vi "ex3.vi"() -> ()   [LabVIEW 2019]
panel:
  in  "stop":bool
  out "Array":bool[](array[boolean])
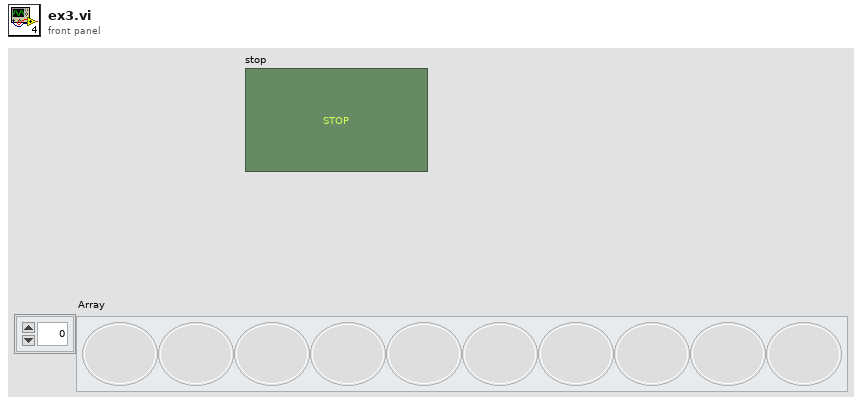
[diagram p1: front panel]
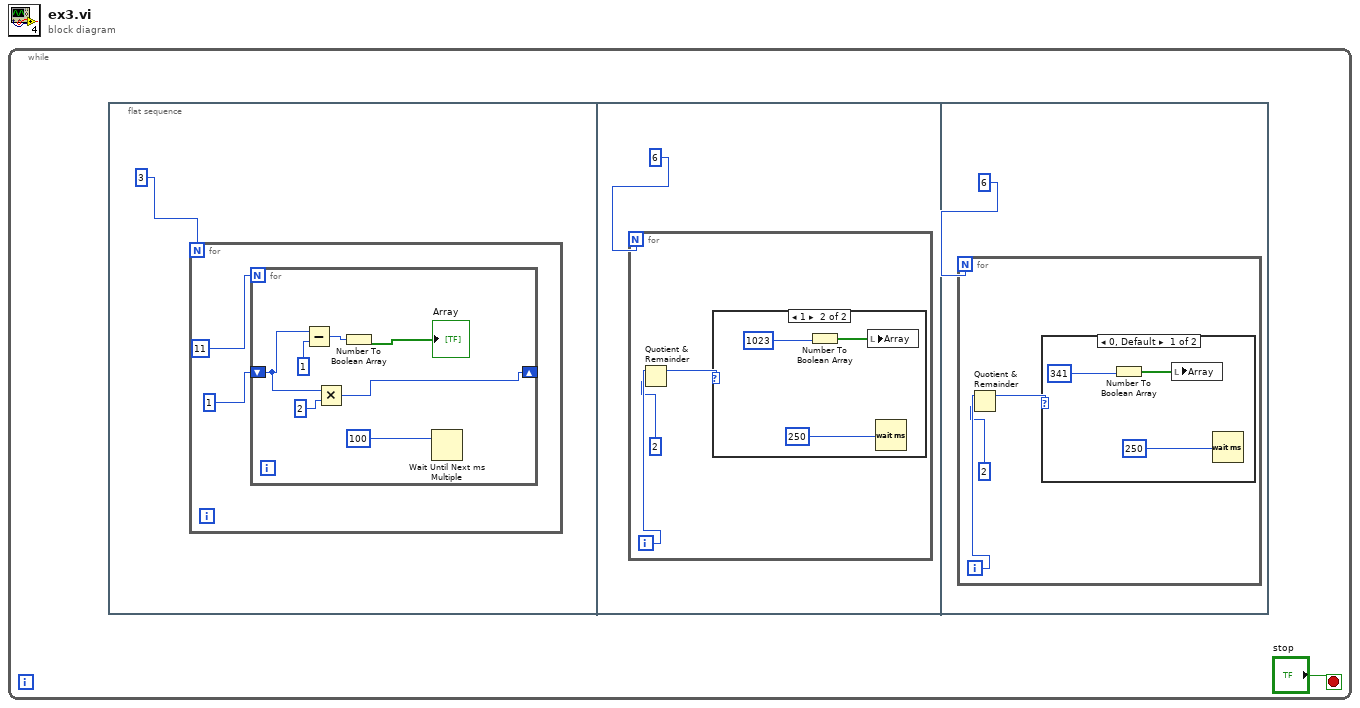
[diagram p0: block diagram]
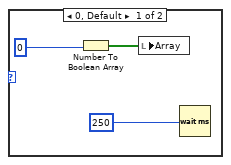
[diagram p2: hidden frame]
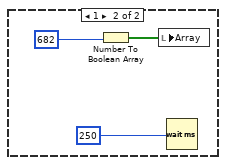
[diagram p3: hidden frame]
diagram:
  n1 = while {
    stop <- "stop" stop-if-true
    n2 = flat-sequence {
      frame #0 {
        n3 = for {
          N: 3 -> [_]
          n4 = for {
            N: 11 -> [_]
            shift-right: [w8] -> _
            shift-left: 1 -> [w5]
            n5 = Subtract(x=w5, y=1) -> (x-y=w7:i32)
            n6 = Multiply(x=w5, y=2) -> (x*y=w8:i32)
            n7 = Number To Boolean Array(number=w7) -> (Boolean array=→"Array":bool[])
            n8 = Wait Until Next ms Multiple(millisecond multiple=100) -> ()  [unwired: 1 out]
          }
        }
      }
      frame #1 {
        n9 = for {
          N: 6 -> [_]
          i -> [w14]
          n10 = Quotient & Remainder(x=w14, y=2) -> (x-y*floor(x/y)=w15:i32)  [unwired: 1 out]
          n11 = case shown="1" w15 {
            frame 0, Default {
              n12 = Number To Boolean Array(number=0) -> (Boolean array=w17:bool[])
              n13 = local write "Array"(w17) -> ()
              n14 = Wait (ms)(milliseconds to wait=250) -> ()  [unwired: 1 out]
            }
            frame 1 {
              n15 = Number To Boolean Array(number=1023) -> (Boolean array=w21:bool[])
              n16 = local write "Array"(w21) -> ()
              n17 = Wait (ms)(milliseconds to wait=250) -> ()  [unwired: 1 out]
            }
          }
        }
      }
      frame #2 {
        n18 = for {
          N: 6 -> [_]
          i -> [w24]
          n19 = Quotient & Remainder(x=w24, y=2) -> (x-y*floor(x/y)=w25:i32)  [unwired: 1 out]
          n20 = case shown="0, Default" w25 {
            frame 0, Default {
              n21 = Number To Boolean Array(number=341) -> (Boolean array=w27:bool[])
              n22 = local write "Array"(w27) -> ()
              n23 = Wait (ms)(milliseconds to wait=250) -> ()  [unwired: 1 out]
            }
            frame 1 {
              n24 = Number To Boolean Array(number=682) -> (Boolean array=w31:bool[])
              n25 = local write "Array"(w31) -> ()
              n26 = Wait (ms)(milliseconds to wait=250) -> ()  [unwired: 1 out]
            }
          }
        }
      }
    }
  }
